vi "Get FrontPanel Ref.vi"(11 "Series UI Actor in":refnum<class "Series UI Actor.lvclass">) -> (2 "FrontPanel Ref":refnum<vi>, 3 "Series UI Actor out":refnum<class "Series UI Actor.lvclass">)   [LabVIEW 2024, in "Series UI Actor.lvlib" / "Series UI Actor.lvclass"]
uses:
  Series UI Actor.lvclass
  Series UI Actor.lvclass/Series UI Actor.ctl
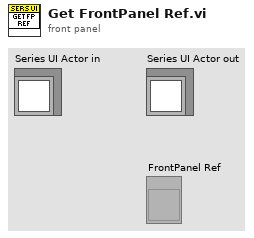
[diagram p1: front panel]
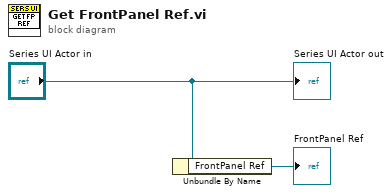
[diagram p0: block diagram]
diagram:
  n1 = Unbundle By Name("Series UI Actor in") -> ("FrontPanel Ref"=→"FrontPanel Ref":refnum<vi>)
  "Series UI Actor out" <- "Series UI Actor in"
